vi "Test App Get Process Throws Error if not found.vi"(8 "error in (no error)":errorcluster, 11 "Application Test In":refnum<class "Application Test.lvclass">) -> (0 "error out":errorcluster, 3 "Application Test Out":refnum<class "Application Test.lvclass">)   [LabVIEW 2020, in "Application Test.lvclass"]
uses:
  Application Test.lvclass
  C:/Program Files (x86)/National Instruments/LabVIEW 2020/vi.lib/Asteme/LUnit/Test Case.lvclass
  Framework/Process/Process.lvclass/Process.ctl
  Framework/Application/Application.lvclass/Application.ctl
  <vilib>/Asteme/LUnit/Test Case.lvclass/Test Case.ctl
  <vilib>/Asteme/LUnit/LUnit Assertion Result.lvclass/LUnit Assertion Result.ctl
  Framework/Process/Protected/Messaging/Request Message.vi
  Framework/Process/Public/Get Lifecycle State.vi
  <vilib>/Asteme/LUnit/Palette/Fail.vi
  <vilib>/Asteme/LUnit/Palette/Pass.vi
  <vilib>/Asteme/LUnit/Set Assertion Type.vi
  Framework/Process/Private/SubVIs/Wait for finish.vi
  Framework/Process/Protected/Messaging/Enqueue Message.vi
  Framework/Process/Private/SubVIs/Set Lifecycle State.vi
  Framework/Process/Private/SubVIs/Enqueue Request Message.vi
  <vilib>/Utility/error.llb/Clear Errors.vi
  <vilib>/Asteme/LUnit/Add test result.vi
  <vilib>/Asteme/LUnit/LUnit Write Passed.vi
  <vilib>/Asteme/LUnit/LUnit Get Test Case.vi
  <vilib>/Asteme/LUnit/LUnit Write Message.vi
  <vilib>/Asteme/LUnit/LUnit Write Description.vi
  <vilib>/Asteme/LUnit/LUnit Write Assertion Type.vi
  <vilib>/Asteme/LUnit/Read Test Case Name.vi
  Framework/Application/Application.lvclass
  C:/Users/anton/Documents/GitHub/Triarc-Framework/source/Framework/Process/Process.lvclass
  <vilib>/Utility/error.llb/Error Cluster From Error Code.vi
  Framework/Process/Private/SubVIs/Wait for Response Message.vi
  <vilib>/Asteme/LUnit/Assertion Result/LUnit Get Test Name.vi
  Framework/Process/Process.lvclass
  <vilib>/Asteme/LUnit/LUnit Assertion Result.lvclass
  <vilib>/Asteme/LUnit/Test Case.lvclass
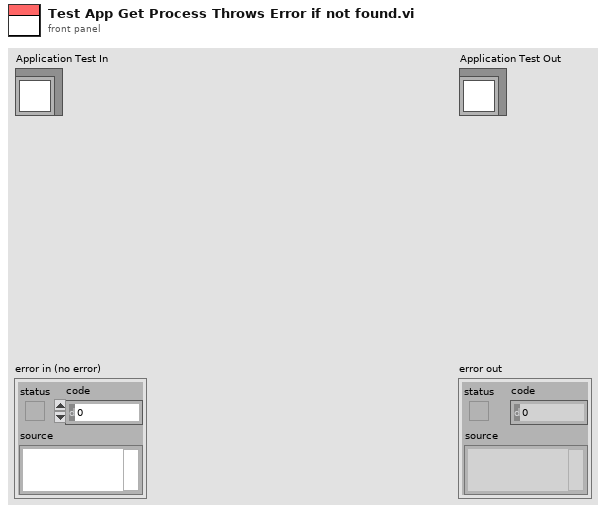
[diagram p1: front panel]
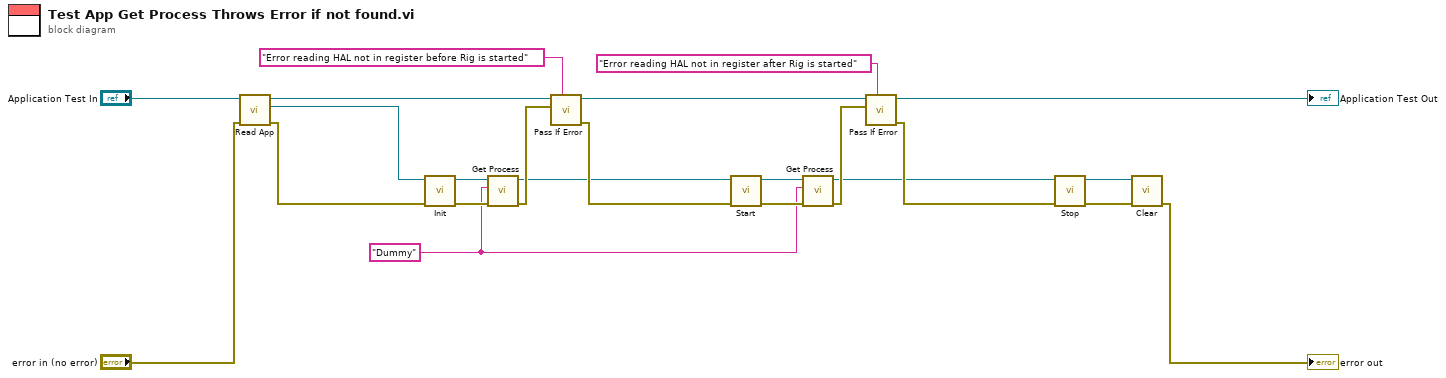
[diagram p0: block diagram]
diagram:
  w4 = "Dummy"
  n1 = call "Read App.vi"("error in (no error)"="error in (no error)", "Application Test In"="Application Test In") -> ("error out"=w21:errorcluster, "App out"=w20:refnum<class "Application.lvclass">, "Application Test Out"=w22:refnum<class "Application Test.lvclass">)  [unwired: 7 in]
  n2 = call-dynamic "Init.vi"("error in (no error)"=w21, "Process In"=w20) -> ("error out"=w12:errorcluster, "Process Out"=w13:refnum<class "Application.lvclass">)  [unwired: 8 in]
  n3 = call "Get Process.vi"("error in (no error)"=w12, "Process Name"=w4, "Rig In"=w13) -> ("error out"=w11:errorcluster, "Rig Out"=w9:refnum<class "Application.lvclass">)  [unwired: 6 in, 1 out]
  n4 = call <vilib>:"Pass If Error.vi"("Description"="Error reading HAL not in register before Rig is started", "Assert error"=w11, "Test Case In"=w22) -> ("error out"=w10:errorcluster, "Test Case Out"=w14:refnum<class "Application Test.lvclass">)  [unwired: 7 in]
  n5 = call "Start.vi"("error in (no error)"=w10, "Process In"=w9) -> ("error out"=w8:errorcluster, "Process Out"=w3:refnum<class "Application.lvclass">)  [unwired: 8 in]
  n6 = call "Get Process.vi"("error in (no error)"=w8, "Process Name"=w4, "Rig In"=w3) -> ("error out"=w7:errorcluster, "Rig Out"=w2:refnum<class "Application.lvclass">)  [unwired: 6 in, 1 out]
  n7 = call <vilib>:"Pass If Error.vi"("Description"="Error reading HAL not in register after Rig is started", "Assert error"=w7, "Test Case In"=w14) -> ("error out"=w6:errorcluster, "Test Case Out"=→"Application Test Out":refnum<class "Application Test.lvclass">)  [unwired: 7 in]
  n8 = call "Stop.vi"("error in (no error)"=w6, "Process In"=w2) -> ("error out"=w17:errorcluster, "Process Out"=w19:refnum<class "Application.lvclass">)  [unwired: 7 in, 1 out]
  n9 = call-dynamic "Clear.vi"("error in (no error)"=w17, "Application In"=w19) -> ("error out"=→"error out":errorcluster)  [unwired: 8 in, 1 out]
